vi "GetControlLabel.vi"(2 "error IO":errorcluster, 3 "Ctl Refnum":refnum<vi>) -> (0 "error out":errorcluster, 1 "Label.Text":string)   [LabVIEW 2021, in "MemberVICreation.lvlib" / "BaseAccessorScripter.lvclass"]
uses:
  <resource>/Framework/Providers/LVClassLibrary/NewAccessors/BaseAccessorScripter/BaseAccessorScripter.lvclass
  <vilib>/Utility/Multibyte/NI_Multibyte Utilities.lvlib
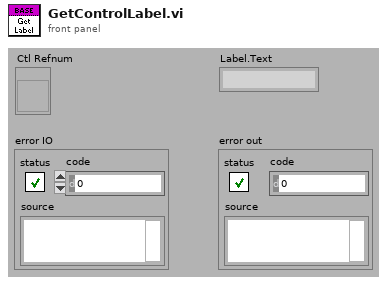
[diagram p1: front panel]
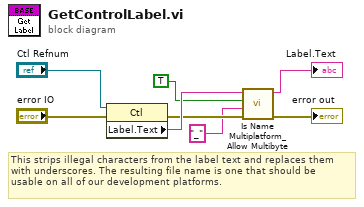
[diagram p0: block diagram]
diagram:
  # "This strips illegal characters from the label text and replaces them\nwith underscores. The resulting file name is one that should be \nusable on all of our development platforms."
  n1 = property class="Ctl"(reference="Ctl Refnum", error in="error IO") -> (error out=w3:errorcluster, "Label.Text"=w6:string)  [unwired: 1 out]
  n2 = call <vilib>:"Is Name Multiplatform_Allow Multibyte.vi"("error in (no error)"=w3, "Replacement"="_", "name must work for all platforms (F)"=TRUE, "filename"=w6) -> ("error out"=→"error out":errorcluster, "suggested filename"=→"Label.Text":string)  [unwired: 4 in, 2 out]
